vi "Engine-New-Window.vi"(8 "error in (no error)":errorcluster, 11 "Window in":refnum<class "Window.lvclass">) -> (0 "error out":errorcluster, 3 "Window out":refnum<class "Window.lvclass">)   [LabVIEW 2020, in "GLF.lvlib" / "Window.lvclass"]
uses:
  Window.lvclass
  C:/Users/saukko/Dev/GLF/Sources/GLF/IAmGLF/IAmGLF.lvclass
  WindowEventInterface/WindowEventInterface.lvclass
  IAmVIEW/IAmVIEW.lvclass
  Window.lvclass/Window.ctl
  C:/Users/saukko/Dev/GLF/Sources/GLF/IUseDVRHandler/IUseDVRHandler.lvclass
  C:/Users/saukko/Dev/GLF/Sources/GLF/Window/Window.lvclass
  <vilib>/Saukko/LV SDL3/Sources/SDL3/Video/WindowID--integer.ctl
  <vilib>/Saukko/LV SDL3/Sources/SDL3/Video/Video.lvlib
  <vilib>/Saukko/LV SDL3/Sources/SDL3/Video/SDL_Window--pointer.ctl
  DVR--cluster.ctl
  IAmGLF/IAmGLF.lvclass
  <vilib>/Saukko/LV SDL3/Sources/SDL3/Render/SDL_Renderer--pointer.ctl
  <vilib>/Saukko/LV SDL3/Sources/SDL3/Render/Render.lvlib
  Flags--cluster.ctl
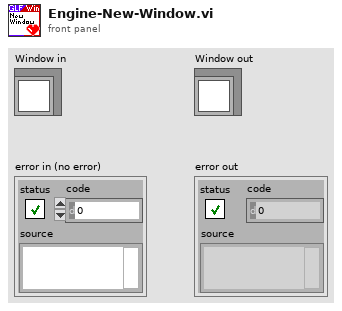
[diagram p1: front panel]
types:
  T1 = typedef "GLF.lvlib/Window.lvclass/DVR--cluster.ctl" = cluster{"SDL_Window *":T2, "Window ID":T3, "SDL_Renderer *":T4, "Event Interface":refnum<class "WindowEventInterface.lvclass">, "VIEW":refnum<class "IAmVIEW.lvclass">, "Flags":T5}
  T2 = typedef "SDL3.lvlib/Video.lvlib/SDL_Window--pointer.ctl" = i64
  T3 = typedef "SDL3.lvlib/Video.lvlib/WindowID--integer.ctl" = u32
  T4 = typedef "SDL3.lvlib/Render.lvlib/SDL_Renderer--pointer.ctl" = i64
  T5 = typedef "GLF.lvlib/Window.lvclass/Flags--cluster.ctl" = cluster{"VIEW Needs Render":bool}
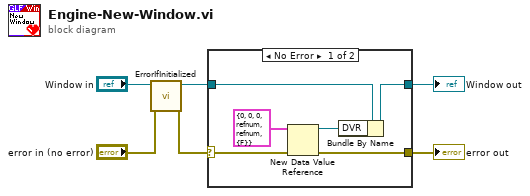
[diagram p0: block diagram]
diagram:
  n1 = call "ErrorIfInitialized.vi"("error in (no error)"="error in (no error)", "IAmGLF in"="Window in") -> ("error out"=w5:errorcluster, "IAmGLF out"=w6:refnum<class "Window.lvclass">)  [unwired: 8 in]
  n2 = case shown="No Error" w5 {
    selector: w5 -> [w10 w14]
    tunnel: [w7 w14] -> w1
    tunnel: [w9 w13] -> w4
    tunnel: w6 -> [w8 w13]
    frame No Error {
      n3 = New Data Value Reference(data value=T1 {"SDL_Window *"=0, "Window ID"=0, "SDL_Renderer *"=0, "Event Interface"=refnum, "VIEW"=refnum, "Flags"={"VIEW Needs Render"=FALSE}} ("DVR"), error in=w10) -> (data value reference=w12:refnum<data-value>, error out=w7:errorcluster)
      n4 = Bundle By Name(cluster=w8, "DVR"=w12) -> (w9:refnum<class "Window.lvclass">)
    }
    frame Error {
    }
  }
  "error out" <- w1
  "Window out" <- w4
